vi "Get Last Value.vi"(11 "array":dbl[](array[numeric])) -> (0 "element":dbl)   [LabVIEW 2025]
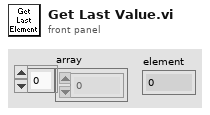
[diagram p1: front panel]
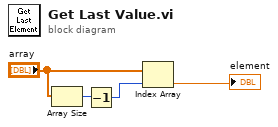
[diagram p0: block diagram]
diagram:
  n1 = Array Size(array="array") -> (size(s)=w3:i32)
  n2 = Decrement(x=w3) -> (x-1=w2:i32)
  n3 = Index Array(array="array", index=w2) -> (element=→"element":dbl)
